vi "DDPCA-300_Set.vi"(10 "Gain Exponent (10^  A/V)":dbl(slide)=4.0 min=4.0 max=13.0 step=1.0 scale=4.0..13.0, 11 "Index":i32) -> (2 "Gain (V/A)":dbl, 3 "Overload":bool)   [LabVIEW 2010]
uses:
  <userlib>/FEMTO/Control/Set_Gain_DDPCA-300.vi
  <userlib>/FEMTO/FEMTO_LUCI-10.lvlib
panel:
  # "Remote Control LUCI-10 DDPCA-300"
  # "Device Information"
  # "DDPCA-300"
  # "Gain Setting"
  # "Overload"
  # "Sophisticated Tools for Signal Recovery"
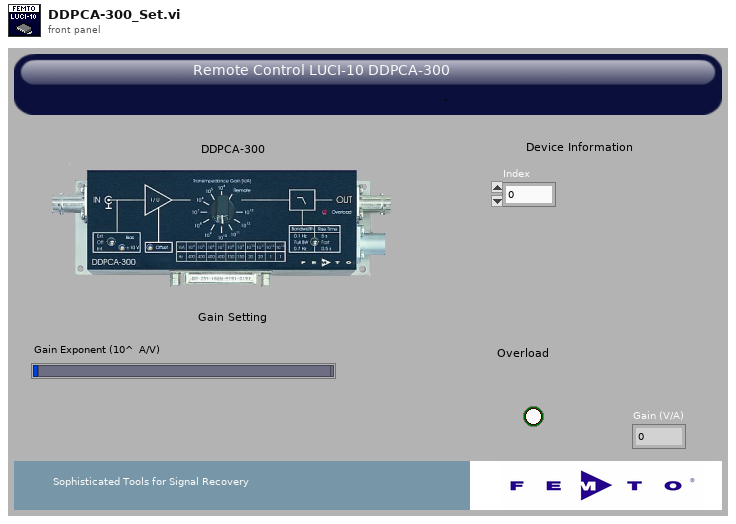
[diagram p1: front panel]
types:
  T1 = enum16{"DDPCA-300", "DLPCA-200", "DHPCA-100", "OE-200", "LIA-MV-150-S", "LIA-MV-150-D", "LIA-MV-200-L", "LIA-MV-200-H", "LIA-MVD-200-L", "LIA-MVD-200-H", "DLPVA-100-BUN-S", "DLPVA-100-BLN-S", "DLPVA-100-B-S", "DLPVA-100-B-D", "DLPVA-100-F-S", "DLPVA-100-F-D", "DHPVA-100", "DHPVA-200", "DUPVA-1-60", "DUPVA-1-70"}
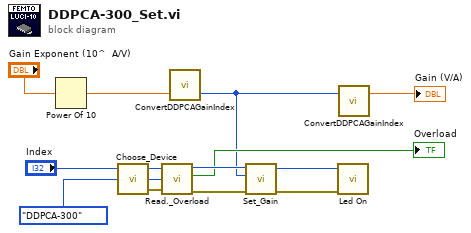
[diagram p0: block diagram]
diagram:
  n1 = Power Of 10(x="Gain Exponent (10^  A/V)") -> (10^x=w5:dbl)
  n2 = call <userlib>:"Choose_Device.vi"("Choose_Device"=T1."DDPCA-300", "Index"="Index") -> ("error out"=w13:errorcluster, "Device_type"=w12:T1, "Index_Out"=w11:i32)  [unwired: 1 in]
  n3 = call <userlib>:"Read._Overload.vi"("Index"=w11, "Choose_Device"=w12, "error in (no error)"=w13) -> ("Index_Out"=w8:i32, "Overload"=→"Overload":bool, "error out"=w9:errorcluster)  [unwired: 1 out]
  n4 = call "ConvertDDPCAGainIndex.vi"("Gain (V/A)"=w5) -> ("Gain (Index)"=w4:i32)  [unwired: 1 in, 1 out]
  n5 = call-poly <userlib>:"Set_Gain.vi"("error in"=w9, "Gain [V/A]"=w4, "index"=w8) -> ("error out"=w1:errorcluster, "index_out"=w2:i32)  [unwired: 1 in, 1 out]
  n6 = call <userlib>:"Led On.vi"("error in (no error)"=w1, "index"=w2) -> ()  [unwired: 7 in, 3 out]
  n7 = call "ConvertDDPCAGainIndex.vi"("Gain (Index)"=w4) -> ("Gain (V/A)"=→"Gain (V/A)":dbl)  [unwired: 1 in, 1 out]
